vi "Ex13.vi"() -> ()   [LabVIEW 2016]
uses:
  <vilib>/Analysis/polynomials.llb/Unique Numbers and Multiplicity (DBL).vi
  <vilib>/Analysis/NI_AALPro.lvlib
panel:
  out "출력 배열 2":dbl[](array[numeric])
  out "출력 배열":dbl[](array[numeric])
  out "웨이브폼 그래프":dbl[][](graph)
  out "최소값":dbl
  out "최대값":dbl
  out "element 2":dbl
  out "배열":dbl[](array[numeric])
  out "element":dbl
  in  "n번째 큰 값":dbl
  in  "n번째 작은 값":dbl
  in  "?":bool
  in  "스위치":bool
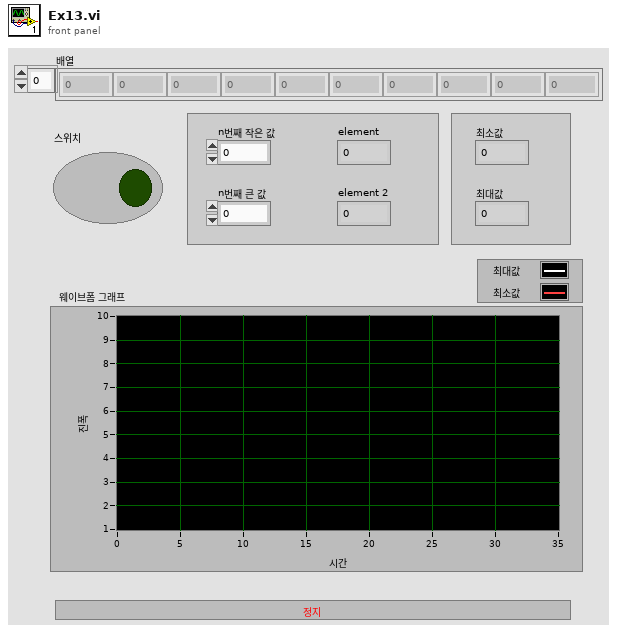
[diagram p1: front panel]
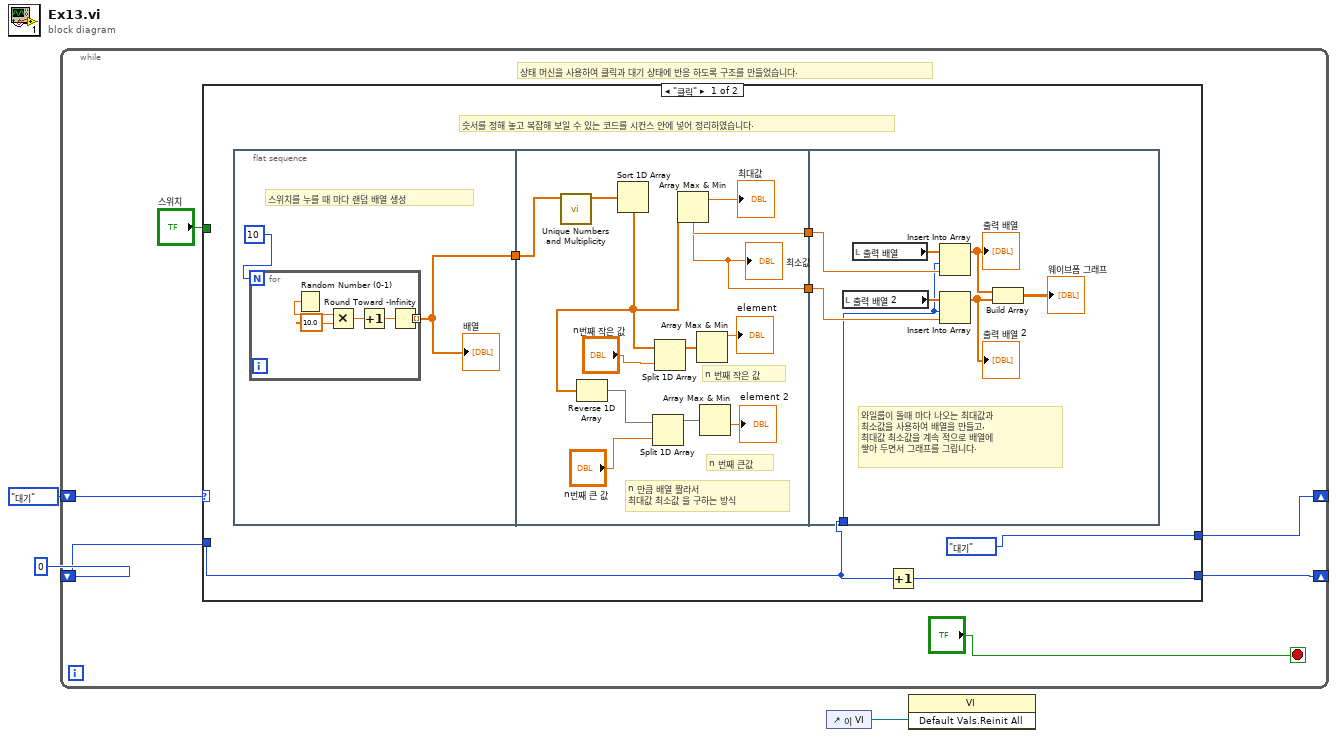
[diagram p0: block diagram]
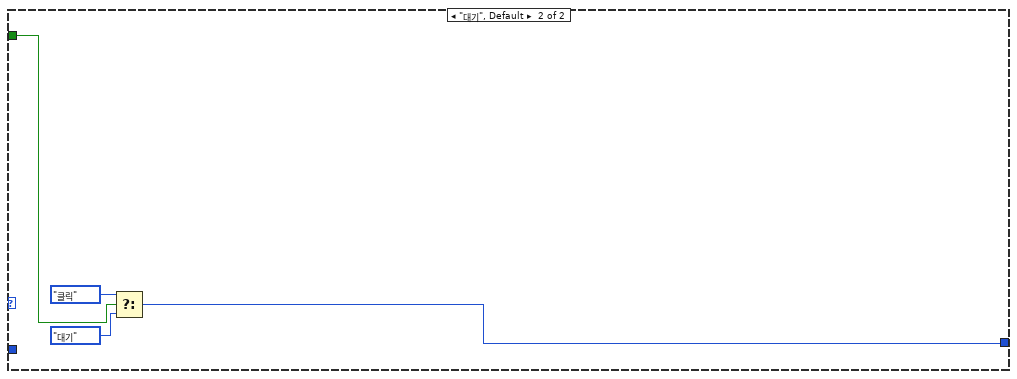
[diagram p2: hidden frame]
diagram:
  n1 = while {
    shift-right: [w6] -> _
    shift-left: enum16{"클릭", "대기"}."대기" -> [w8]
    shift-right: [w4] -> _
    shift-left: 0 -> [w5]
    stop <- "?" stop-if-true
    # "상태 머신을 사용하여 클릭과 대기 상태에 반응 하도록 구조를 만들었습니다."
    n2 = case shown="\"클릭\"" w8 {
      tunnel: "스위치" -> [_ w44]
      tunnel: [enum16{"클릭", "대기"}."대기" w43] -> w6
      tunnel: w5 -> [w11 _]
      tunnel: [w13 _] -> w4
      frame "클릭" {
        # "숫서를 정해 놓고 복잡해 보일 수 있는 코드를 시컨스 안에 넣어 정리하였습니다."
        n3 = flat-sequence {
          tunnel: [w16] -> w14
          tunnel: w14 -> [w32]
          tunnel: [w25] -> w12
          tunnel: [w24] -> w10
          tunnel: w11 -> [w38]
          tunnel: w12 -> [w42]
          tunnel: w10 -> [w39]
          frame #0 {
            # "스위치를 누를 때 마다 랜덤 배열 생성"
            n4 = for {
              N: 10 -> [_]
              tunnel: [w18] -> w16 mode=indexing
              n5 = Random Number (0-1)() -> (number: 0 to 1=w22:dbl)
              n6 = Multiply(x=w22, y=10.0) -> (x*y=w20:dbl)
              n7 = Increment(x=w20) -> (x+1=w19:dbl)
              n8 = Round Toward -Infinity(1:w19) -> (0:w18:dbl)
            }
            "배열" <- w16
          }
          frame #1 {
            # "n 만큼 배열 짤라서\n최대값 최소값 을 구하는 방식"
            # "n 번째 큰값"
            # "n 번째 작은 값"
            n9 = call-poly <vilib>:"Unique Numbers and Multiplicity.vi"("Numbers"=w32) -> ("Unique Numbers"=w31:dbl[])  [unwired: 8 in, 2 out]
            n10 = Sort 1D Array(array=w31) -> (sorted array=w26:dbl[])
            n11 = Reverse 1D Array(array=w26) -> (reversed array=w30:dbl[])
            n12 = Split 1D Array(array=w30, index="n번째 큰 값") -> (first subarray=w28:dbl[])  [unwired: 1 out]
            n13 = Split 1D Array(array=w26, index="n번째 작은 값") -> (first subarray=w34:dbl[])  [unwired: 1 out]
            n14 = Array Max & Min(array=w26) -> (max value=w25:dbl, min value=w24:dbl)  [unwired: 2 out]
            "최대값" <- w25
            "최소값" <- w24
            n15 = Array Max & Min(array=w34) -> (max value=→"element":dbl)  [unwired: 3 out]
            n16 = Array Max & Min(array=w28) -> (min value=→"element 2":dbl)  [unwired: 3 out]
          }
          frame #2 {
            # "와일룹이 돌때 마다 나오는 최대값과 \n최소값을 사용하여 배열을 만들고, \n최대값 최소값을 계속 적으로 배열에 \n쌓아 두면서 그래프를 그립니다."
            n17 = local read "출력 배열 2"() -> (w40:dbl[])
            n18 = local read "출력 배열"() -> (w41:dbl[])
            n19 = Insert Into Array(array=w41, index=w38, new element=w42) -> (w37:dbl[])
            "출력 배열" <- w37
            n20 = Insert Into Array(array=w40, index=w38, new element=w39) -> (w36:dbl[])
            "출력 배열 2" <- w36
            n21 = Build Array(w37, w36) -> (→"웨이브폼 그래프":dbl[][])
          }
        }
        n22 = Increment(x=w11) -> (x+1=w13:i32)
      }
      frame "대기", Default {
        n23 = Select(t=enum16{"클릭", "대기"}."클릭", s=w44, f=enum16{"클릭", "대기"}."대기") -> (s? t:f=w43:enum16{"클릭", "대기"})
      }
    }
  }
  n24 = control-ref of="이 VI"() -> (w1:refnum<vi>)
  n25 = invoke class="VI" method="Default Vals.Reinit All"(reference=w1) -> ()  [unwired: 2 in, 3 out]
